vi "MasterAquisitionFile_2P.vi"() -> ()   [LabVIEW 2017]
uses:
  <vilib>/userdefined/High Color/IMAQdx.ctl
  <vilib>/vision/driver/IMAQdx.llb/IMAQdx Camera Control Mode.ctl
  <vilib>/vision/driver/IMAQdx.llb/IMAQdx Acquisition Mode.ctl
  <vilib>/vision/driver/IMAQdx.llb/IMAQdx Buffer Number Mode.ctl
  <vilib>/DAQmx/miscellaneous.llb/DAQmx Fill In Error Info.vi
  <vilib>/DAQmx/read.llb/DAQmx Read (Digital 1D Bool 1Chan 1Samp).vi
  <vilib>/DAQmx/create/channels.llb/DAQmx Create Channel (DI-Digital Input).vi
  <vilib>/DAQmx/create/channels.llb/DAQmx Create Channel (DO-Digital Output).vi
  <vilib>/DAQmx/read.llb/DAQmx Read (Analog 1D Wfm NChan NSamp).vi
  <vilib>/DAQmx/configure/trigger.llb/DAQmx Start Trigger (Digital Edge).vi
  <vilib>/DAQmx/configure/timing.llb/DAQmx Timing (Sample Clock).vi
  <vilib>/DAQmx/create/channels.llb/DAQmx Create Channel (AI-Voltage-Basic).vi
  <vilib>/DAQmx/configure/timing.llb/DAQmx Timing (Implicit).vi
  <vilib>/DAQmx/create/channels.llb/DAQmx Create Channel (CO-Pulse Generation-Frequency).vi
  <vilib>/DAQmx/write.llb/DAQmx Write (Digital 1D Bool NChan 1Samp 1Line).vi
  <vilib>/vision/driver/NI_Vision_Acquisition_Software.lvlib
  <resource>/objmgr/imaqdx.rc
panel:
  in  "stop":bool
  in  "Offset (s)":dbl=15.0
  in  "Duration (s)":dbl=0.1 step=0.1
  in  "Interval (s)":dbl=30.0
  out "Solenoids":bool[](array[boolean])
  in  "Left Pad Solenoid":tag="Dev1/port0/line5"
  in  "Right Pad Solenoid":tag="Dev1/port0/line6"
  in  "Auditory Solenoid":tag="Dev1/port0/line7"
  in  "RPad":dbl=1.0
  in  "LPad":dbl=1.0
  in  "Aud":dbl=1.0
  out "?":T1(plugin-control)
  out "Web Cam Fs":dbl(knob) scale=0.0..200.0
  out "Web Cam":bool
  in  "WebCam ID":T2="cam2"
  out "Complete":bool
  out "Whisk Cam":bool
  out "Analog":bool
  out "MScan Trig":bool
  in  "MScan Trigger":tag="Dev1/port0/line3"
  out "?":bool[](array[boolean])
  out "Hexadecimal Data":u32 format="%x"
  out "Time Elapsed (Min)":cluster{dbl, dbl}(slide)={16.0, 0.0} scale=0.0..16.0 scale format="%#_2g"
  out "Whisker Camera":bool=TRUE
  out "Analog Data":bool
  out "Analog Samples":i32
  in  "Analog Channel Labels":string[](array[string])=["Force_Sensor", "Force_Sensor", "Solenoid_LeftPad", "Solenoid_RightPad", "Solenoid_Auditory", "Respiration", "EMG", "Neural_RH"]
  in  "Analog Input Channels":tag="Dev1/ai2"
  in  "Whisker Cam ID":T2="cam1"
  in  "?":cluster{"Analog Fs":u16}={"Analog Fs"=20000} {"Analog Fs" format="%0.0f"}
  in  "?":cluster{"WhiskerCam Fs":u16}={"WhiskerCam Fs"=150}
  out "Notes Size":i32=7
  out "Notes Reversed":string[](array[string])=["Experimenter", "Animal ID", "Isoflurane time", "Amplifier Gain", "Session ID", "Hemisphere", "Solenoid PSI"]
  out "Notes Array":string[](array[string])=["Solenoid PSI", "Hemisphere", "Session ID", "Amplifier Gain", "Isoflurane time", "Animal ID", "Experimenter"]
  in  "Notes:":T3={"Experimenter"="0\n", "Animal ID"="", "Isoflurane time"="", "Amplifier Gain"="", "Session ID"="", "Hemisphere"="", "Solenoid PSI"=""}
  in  "Whisk Cam Trigger":tag="Dev1/ctr0"
  in  "Target Path":path=path "C:/Users/klt8/Documents" caption="Final Saved File Location"
  out "Dropped":u32(slide) caption="Whisk Cam" scale=0.0..50.0
  out "Current File Name":string="190410_10_32_56"
  in  "Time (min)":dbl(knob)=16.0 min=0.5 max=20.0 step=0.5 scale=0.0..20.0 scale format="%#_3g"
  in  "Temp Path":path=path "C:/LabVIEW Temp Files" caption="Temporary File Path"
  out "Last Whisk Buffer":u32=45000
  out "Whisk Cam Fs":dbl(knob) scale=0.0..200.0 scale format="%#1_6g"
  # "LPad Sol"
  # "RPad Sol"
  # "Aud Sol"
  # "Web Cam ID"
  # "Whisk Cam ID"
  # "AnalogFs"
  # "WhiskFs"
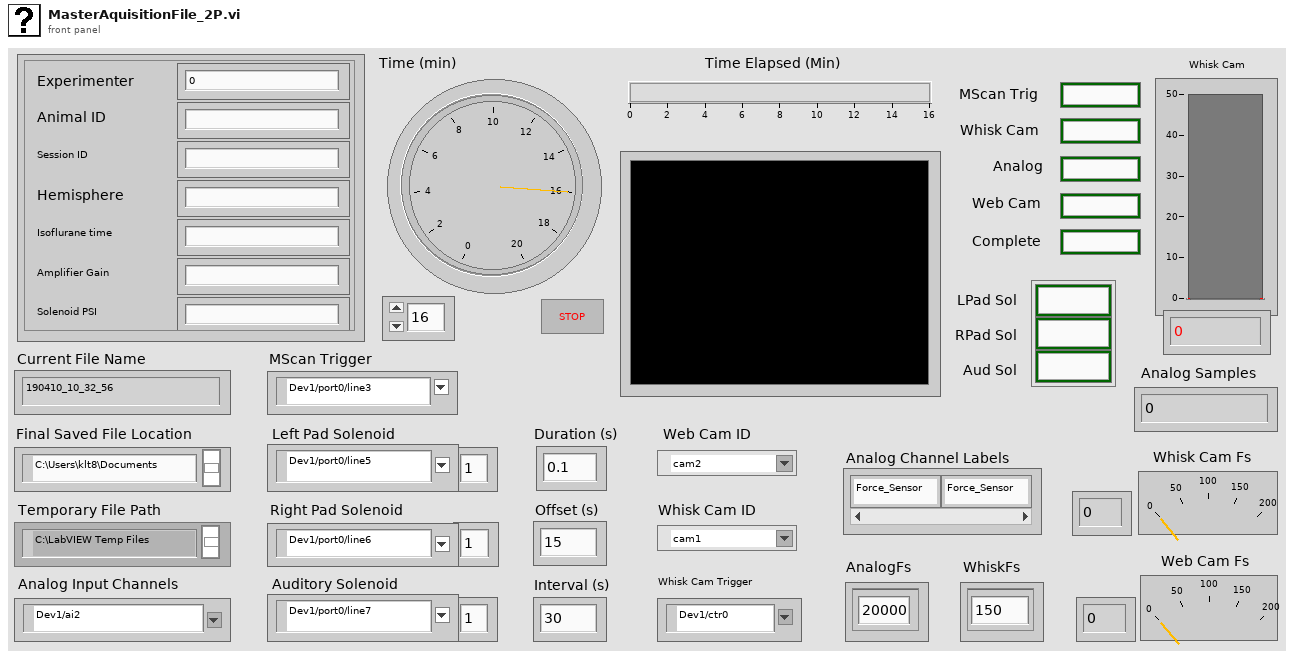
[diagram p1: front panel]
types:
  T1 = typedef "IMAQ Image.ctl" = refnum<image>
  T2 = typedef "IMAQdx.ctl" = refnum<k21>
  T3 = cluster{"Experimenter":string, "Animal ID":string, "Isoflurane time":string, "Amplifier Gain":string, "Session ID":string, "Hemisphere":string, "Solenoid PSI":string}
  T4 = enum16{"open", "open or create", "create or replace", "create", "open (read-only)"}
  T5 = typedef "NI_Vision_Acquisition_Software.lvlib/IMAQdx Camera Control Mode.ctl" = enum32{"Controller", "Listener"}
  T6 = enum16{"open", "replace", "create", "open or create", "replace or create", "replace or create with confirmation"}
  T7 = typedef "NI_Vision_Acquisition_Software.lvlib/IMAQdx Acquisition Mode.ctl" = enum32{"One Shot", "Continuous"}
  T8 = enum16{"big-endian, network order", "native, host order", "little-endian"}
  T9 = typedef "NI_Vision_Acquisition_Software.lvlib/IMAQdx Buffer Number Mode.ctl" = enum32{"Next", "Last", "Buffer Number", "Every", "Last New"}
  T10 = typedef "Image Type" = u32
  T11 = typedef "IMAQ AVI2 Refnum.ctl" = refnum<k20>
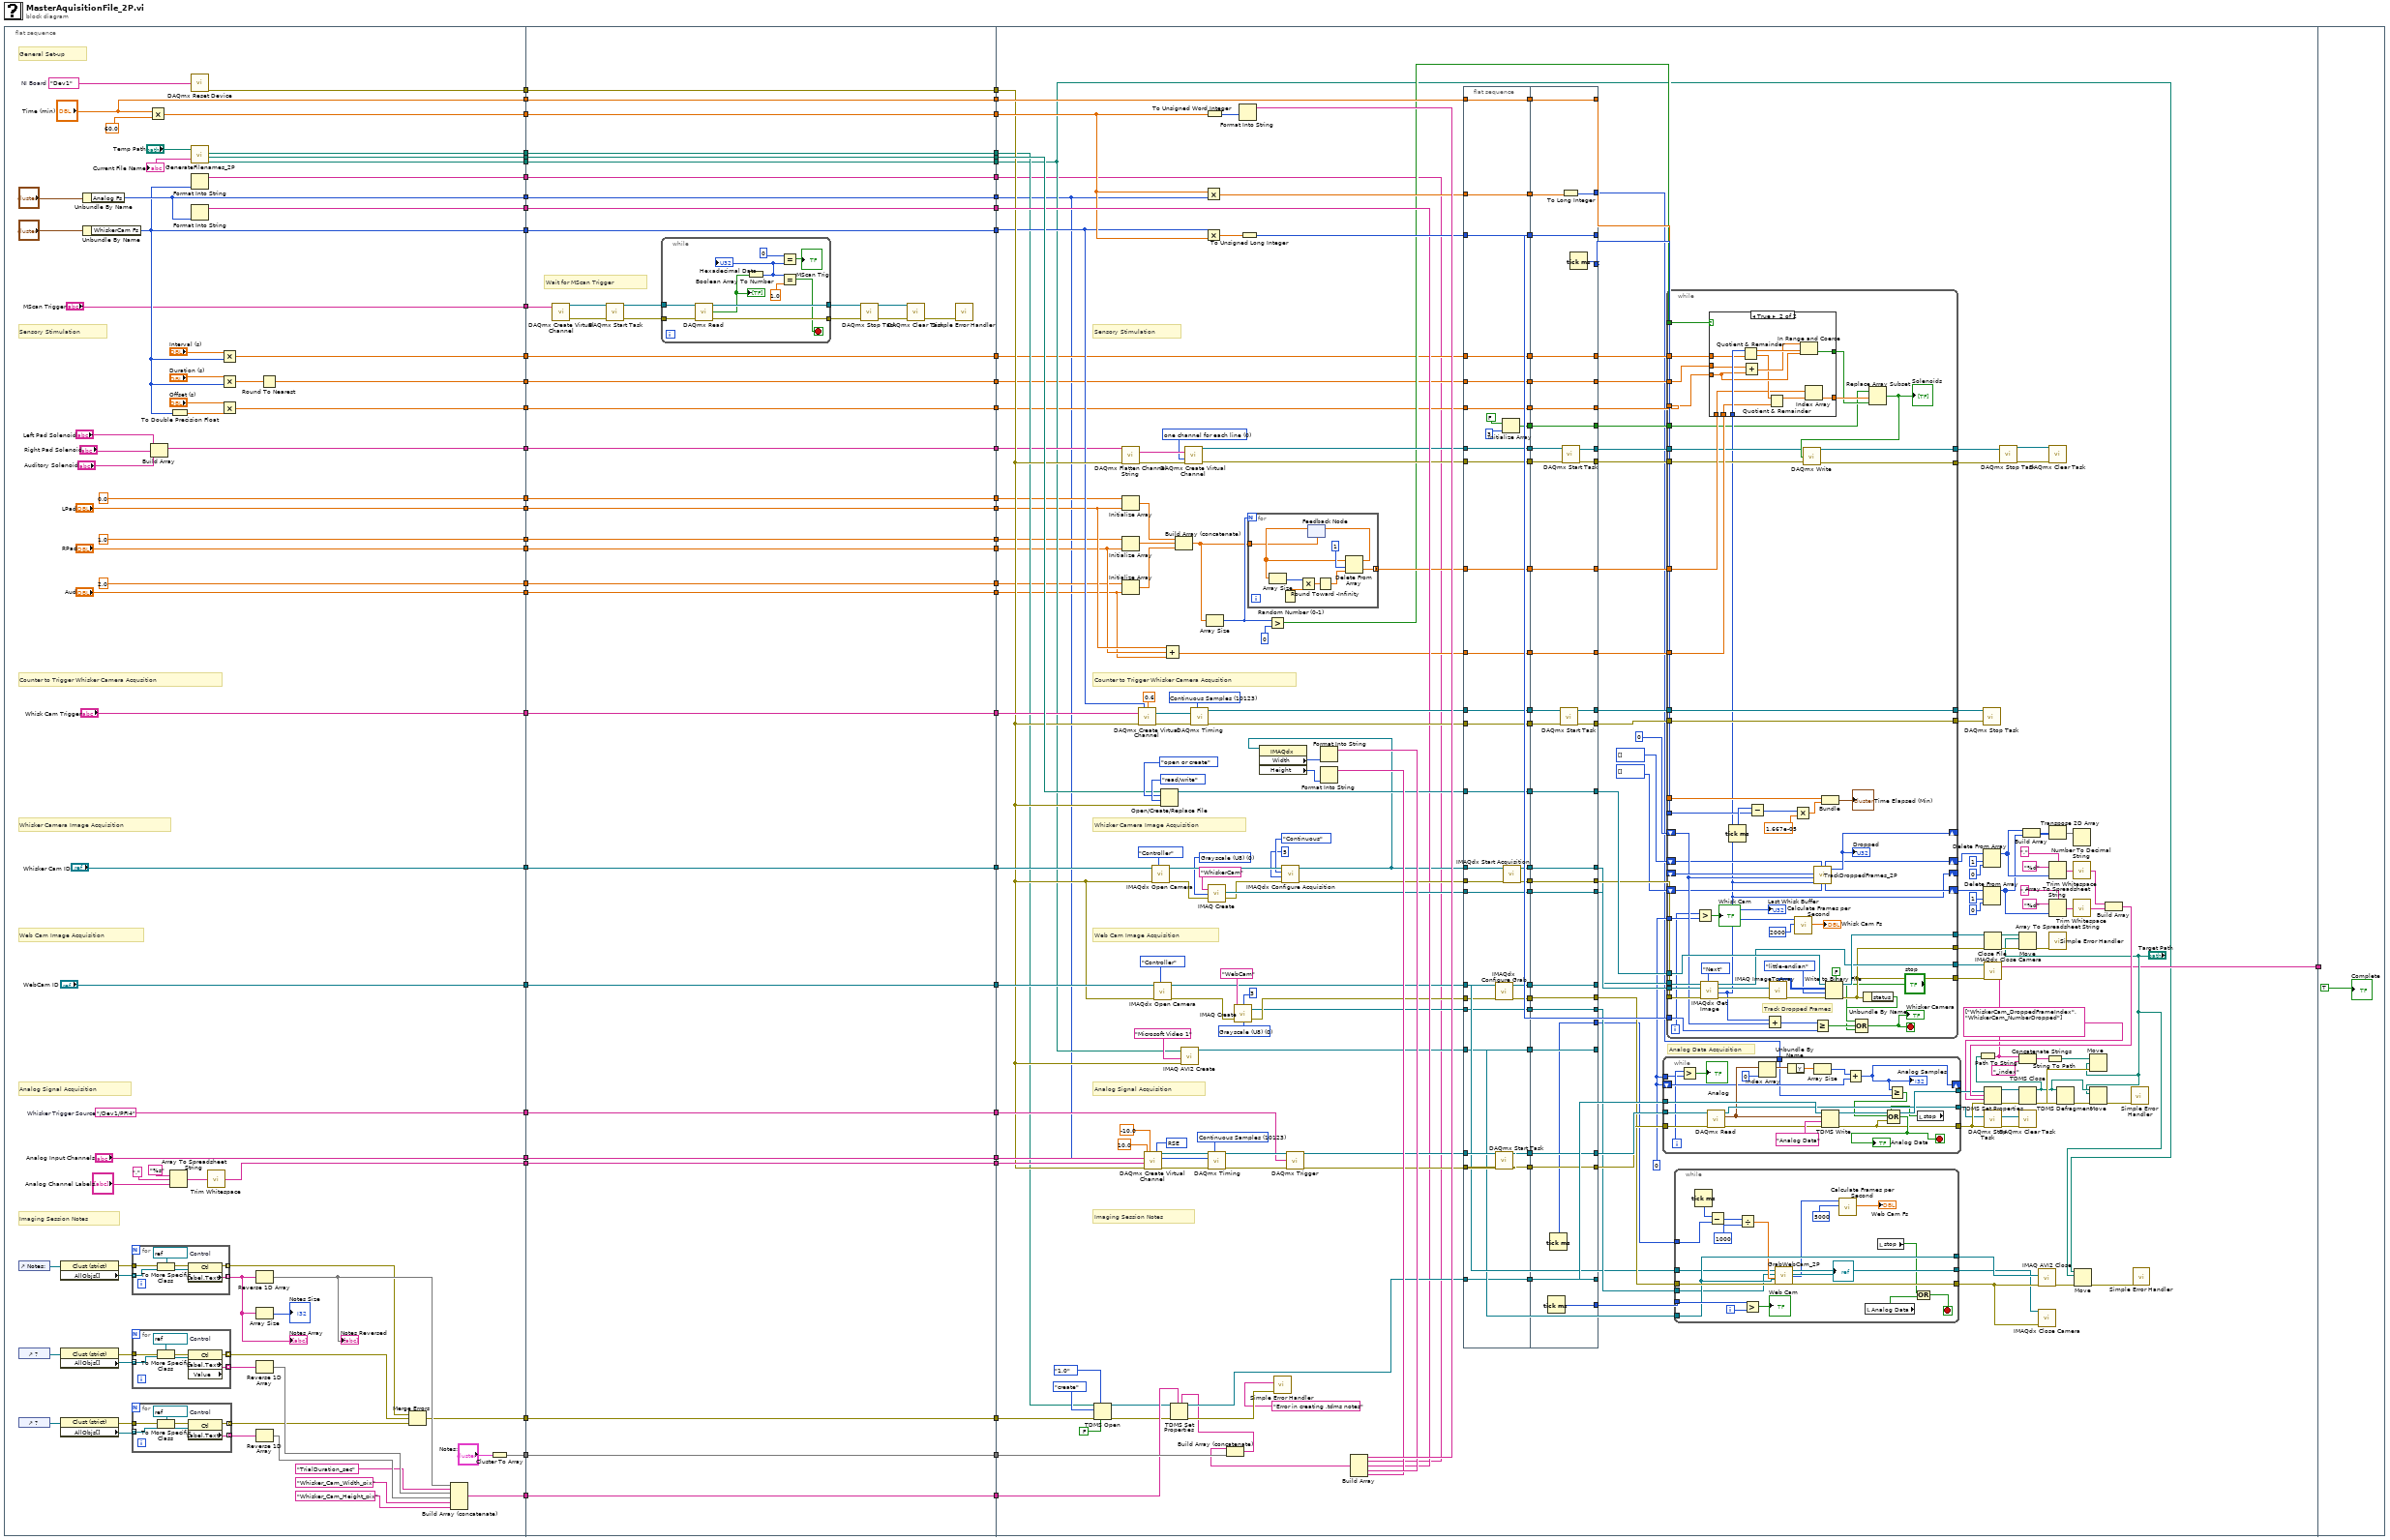
[diagram p0: block diagram]
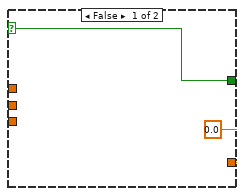
[diagram p2: hidden frame]
diagram:
  n1 = flat-sequence {
    tunnel: [w100] -> w45
    tunnel: [w99] -> w44
    tunnel: ["Time (min)"] -> w43
    tunnel: [w97] -> w42
    tunnel: [w96] -> w41
    tunnel: [w95] -> w40
    tunnel: [w94] -> w39
    tunnel: [w93] -> w38
    tunnel: ["Whisk Cam Trigger"] -> w37
    tunnel: [w91] -> w36
    tunnel: ["Analog Input Channels"] -> w35
    tunnel: ["Whisker Cam ID"] -> w34
    tunnel: [w88] -> w33
    tunnel: [w84] -> w32
    tunnel: [w87] -> w31
    tunnel: ["WebCam ID"] -> w29
    tunnel: ["MScan Trigger"] -> w28
    tunnel: [w81] -> w27
    tunnel: [w80] -> w24
    tunnel: [w79] -> w23
    tunnel: [w75] -> w19
    tunnel: [w70] -> w15
    tunnel: [w69] -> w14
    tunnel: [w68] -> w13
    tunnel: [1.0 ("element")] -> w6
    tunnel: [0.0 ("element")] -> w5
    tunnel: [2.0 ("element")] -> w4
    tunnel: ["Aud"] -> w3
    tunnel: ["RPad"] -> w2
    tunnel: ["LPad"] -> w1
    tunnel: [w168] -> w60
    tunnel: [w180] -> w59
    tunnel: [w181] -> w58
    tunnel: [w182] -> w57
    tunnel: [w183] -> w56
    tunnel: [w170] -> w55
    tunnel: [w184] -> w54
    tunnel: [w169] -> w53
    tunnel: [w185] -> w52
    tunnel: [w186] -> w51
    tunnel: [w187] -> w50
    tunnel: [w188] -> w49
    tunnel: [w189] -> w48
    tunnel: [w190] -> w47
    tunnel: [w191] -> w46
    tunnel: w45 -> [w191]
    tunnel: w44 -> [w190]
    tunnel: w43 -> [w189]
    tunnel: w42 -> [w188]
    tunnel: w41 -> [w187]
    tunnel: w40 -> [w186]
    tunnel: w39 -> [w185]
    tunnel: w38 -> [w169]
    tunnel: w37 -> [w184]
    tunnel: w36 -> [w170]
    tunnel: w35 -> [w183]
    tunnel: w34 -> [w182]
    tunnel: w33 -> [w181]
    tunnel: w32 -> [w180]
    tunnel: w31 -> [w168]
    tunnel: [w166] -> w30
    tunnel: w29 -> [w166]
    tunnel: w28 -> [w167]
    tunnel: w27 -> [w165]
    tunnel: [w165] -> w26
    tunnel: w24 -> [w164]
    tunnel: w23 -> [w163]
    tunnel: [w164] -> w22
    tunnel: [w163] -> w21
    tunnel: [w162] -> w20
    tunnel: w19 -> [w162]
    tunnel: [w161] -> w18
    tunnel: [w159] -> w17
    tunnel: [w160] -> w16
    tunnel: w15 -> [w161]
    tunnel: w14 -> [w160]
    tunnel: w13 -> [w159]
    tunnel: [w153] -> w12
    tunnel: [w154] -> w11
    tunnel: [w155] -> w10
    tunnel: [w158] -> w9
    tunnel: [w157] -> w8
    tunnel: [w156] -> w7
    tunnel: w6 -> [w158]
    tunnel: w5 -> [w157]
    tunnel: w4 -> [w156]
    tunnel: w3 -> [w155]
    tunnel: w2 -> [w154]
    tunnel: w1 -> [w153]
    tunnel: w60 -> [w297]
    tunnel: w59 -> [w307]
    tunnel: w58 -> [w256]
    tunnel: w57 -> [w306]
    tunnel: w56 -> [w305]
    tunnel: w55 -> [w304]
    tunnel: w54 -> [w303]
    tunnel: w53 -> [w302]
    tunnel: w52 -> [w240]
    tunnel: w51 -> [w206]
    tunnel: w50 -> [w301]
    tunnel: w49 -> [w205]
    tunnel: w48 -> [w292]
    tunnel: w47 -> [w300]
    tunnel: w46 -> [w299]
    tunnel: w30 -> [w283]
    tunnel: w26 -> [w218]
    tunnel: [w229] -> w25
    tunnel: w22 -> [w224]
    tunnel: w21 -> [w222]
    tunnel: w20 -> [w219]
    tunnel: w18 -> [w217]
    tunnel: w17 -> [w208]
    tunnel: w16 -> [w216]
    tunnel: w12 -> [w215]
    tunnel: w11 -> [w214]
    tunnel: w10 -> [w213]
    tunnel: w9 -> [w212]
    tunnel: w8 -> [w211]
    tunnel: w7 -> [w210]
    tunnel: w25 -> [_]
    frame #0 {
      w100 = tag "/Dev1/PFI4"  # Whisker Trigger Source
      w104 = tag "Dev1"  # NI Board
      # "Sensory Stimulation"
      # "General Set-up"
      # "Whisker Camera Image Acquisition"
      # "Imaging Session Notes"
      # "Counter to Trigger Whisker Camera Acqusition"
      # "Web Cam Image Acquisition"
      # "Analog Signal Acquisition"
      n2 = control-ref of="Notes:"() -> (w117:refnum<vi>)
      n3 = control-ref of="?"() -> (w115:refnum<vi>)
      n4 = control-ref of="?"() -> (w108:refnum<vi>)
      n5 = property class="Clust (strict)"(reference=w117) -> (error out=w116:errorcluster, "AllObjs[]"=w118:refnum<vi>[])  [unwired: 1 in, 1 out]
      n6 = property class="Clust (strict)"(reference=w115) -> (error out=w113:errorcluster, "AllObjs[]"=w114:refnum<vi>[])  [unwired: 1 in, 1 out]
      n7 = property class="Clust (strict)"(reference=w108) -> (error out=w109:errorcluster, "AllObjs[]"=w111:refnum<vi>[])  [unwired: 1 in, 1 out]
      n8 = Unbundle By Name("?") -> ("Analog Fs"=w95:u16)
      n9 = Unbundle By Name("?") -> ("WhiskerCam Fs"=w94:u16)
      n10 = for {
        tunnel: [w136] -> w123 mode=indexing
        tunnel: w118 -> [w135] mode=indexing
        tunnel: w116 -> [w134]
        tunnel: [w132] -> w122 mode=indexing
        w137 = refnum<vi> refnum  # Control
        n11 = To More Specific Class(target class=w137, reference=w135, error in=w134) -> (specific class reference=w138:refnum<vi>, error out=w133:errorcluster)
        n12 = property class="Ctl"(reference=w138, error in=w133) -> (error out=w132:errorcluster, "Label.Text"=w136:string)  [unwired: 1 out]
      }
      "Notes Array" <- w123
      n13 = for {
        tunnel: [w143] -> w112 mode=indexing
        tunnel: w114 -> [w142] mode=indexing
        tunnel: w113 -> [w141]
        tunnel: [w139] -> w121 mode=indexing
        w144 = refnum<vi> refnum  # Control
        n14 = To More Specific Class(target class=w144, reference=w142, error in=w141) -> (specific class reference=w145:refnum<vi>, error out=w140:errorcluster)
        n15 = property class="Ctl" props=["Label", "Text", "Value"](reference=w145, error in=w140) -> (error out=w139:errorcluster, "Label.Text"=w143:string)  [unwired: 2 out]
      }
      n16 = for {
        tunnel: [w150] -> w110 mode=indexing
        tunnel: w111 -> [w149] mode=indexing
        tunnel: w109 -> [w148]
        tunnel: [w146] -> w120 mode=indexing
        w151 = refnum<vi> refnum  # Control
        n17 = To More Specific Class(target class=w151, reference=w149, error in=w148) -> (specific class reference=w152:refnum<vi>, error out=w147:errorcluster)
        n18 = property class="Ctl"(reference=w152, error in=w147) -> (error out=w146:errorcluster, "Label.Text"=w150:string)  [unwired: 1 out]
      }
      n19 = Multiply(x="Time (min)", y=60.0) -> (x*y=w99:dbl)
      n20 = Build Array("Left Pad Solenoid", "Right Pad Solenoid", "Auditory Solenoid") -> (w75:tag[])
      n21 = Array To Spreadsheet String(delimiter (Tab)=",", array="Analog Channel Labels", 3:"%s" ("format string")) -> (spreadsheet string=w125:string)
      n22 = To Double Precision Float(number=w94) -> (double precision float=w74:dbl)
      n23 = call <vilib>:"DAQmx Reset Device.vi"("device in"=w104) -> ("error out"=w88:errorcluster)  [unwired: 14 in]
      n24 = call "GenerateFilenames_2P.vi"("path"="Temp Path") -> ("Analog file name"=→"Current File Name":string, "TDMS Path"=w79:path, "Basler Path"=w84:path, "WebCam Path"=w81:path)  [unwired: 6 in]
      n25 = Format Into String(w94) -> (resulting string=w97:string)  [unwired: 3 in, 1 out]
      n26 = Format Into String(w95) -> (resulting string=w96:string)  [unwired: 3 in, 1 out]
      n27 = call <vilib>:"Trim Whitespace.vi"("string"=w125) -> ("trimmed string"=w91:string)  [unwired: 1 in]
      n28 = Multiply(x="Interval (s)", y=w94) -> (x*y=w68:dbl)
      n29 = Multiply(x="Duration (s)", y=w94) -> (x*y=w67:dbl)
      n30 = Multiply(x="Offset (s)", y=w74) -> (x*y=w70:dbl)
      n31 = Reverse 1D Array(array=w123) -> (reversed array=w124:string[])
      "Notes Reversed" <- w124
      n32 = Array Size(array=w123) -> (size(s)=→"Notes Size":i32)
      n33 = Reverse 1D Array(array=w112) -> (reversed array=w130:string[])
      n34 = Reverse 1D Array(array=w110) -> (reversed array=w131:string[])
      n35 = Round To Nearest(number=w67) -> (nearest integer value=w69:dbl)
      n36 = Merge Errors(w122, w121, w120) -> (w80:errorcluster)
      n37 = Build Array (concatenate)(w124, "TrialDuration_sec", w130, w131, "Whisker_Cam_Width_pix", "Whisker_Cam_Height_pix") -> (w87:string[])
      n38 = Cluster To Array(cluster="Notes:") -> (array=w93:string[])
    }
    frame #1 {
      # "Wait for MScan Trigger"
      n39 = call-poly <vilib>:"DAQmx Create Virtual Channel.vi"("lines"=w167) -> ("task out"=w175:refnum<k21>, "error out"=w176:errorcluster)  [unwired: 13 in]
      n40 = call <vilib>:"DAQmx Start Task.vi"("task/channels in"=w175, "error in"=w176) -> ("task out"=w179:refnum<k21>, "error out"=w178:errorcluster)  [unwired: 12 in]
      n41 = while {
        tunnel: w179 -> [w201]
        tunnel: w178 -> [w200]
        tunnel: [w198] -> w173
        tunnel: [w199] -> w174
        stop <- w193 stop-if-true
        n42 = call-poly <vilib>:"DAQmx Read.vi"("task/channels in"=w201, "error in"=w200) -> ("task out"=w199:refnum<k21>, "data"=w197:bool[], "error out"=w198:errorcluster)  [unwired: 11 in]
        "?" <- w197
        n43 = Boolean Array To Number(Boolean array=w197) -> (number=w192:u32)
        "Hexadecimal Data" <- w192
        n44 = Equal?(x=w192, y=u32 0) -> (x = y?=→"MScan Trig":bool)
        n45 = Equal?(x=w192, y=1.0) -> (x = y?=w193:bool)
      }
      n46 = call <vilib>:"DAQmx Stop Task.vi"("task/channels in"=w174, "error in"=w173) -> ("task out"=w172:refnum<k21>, "error out"=w171:errorcluster)  [unwired: 12 in]
      n47 = call <vilib>:"DAQmx Clear Task.vi"("task in"=w172, "error in"=w171) -> ("error out"=w177:errorcluster)  [unwired: 13 in]
      n48 = call <vilib>:"Simple Error Handler.vi"("error in (no error)"=w177) -> ()  [unwired: 4 in, 5 out]
    }
    frame #2 {
      w209 = 0 items=["one channel for each line", "one channel for all lines"] ("line grouping")
      w287 = T10 0 items=["Grayscale (U8)", "Grayscale (I16)", "Grayscale (SGL)", "Complex (CSG)", "RGB (U32)", "HSL (U32)", "RGB (U64)", "Grayscale (U16)"] ("Image Type")
      w271 = u32 0 ("y")
      w316 = 10123 items=["Finite Samples"=10178, "Continuous Samples"=10123, "Hardware Timed Single Point"=12522] ("sample mode")
      w315 = 10083 items=["default"=-1, "RSE"=10083, "NRSE"=10078, "Differential"=10106, "Pseudodifferential"=12529] ("input terminal configuration")
      w317 = 10123 items=["Finite Samples"=10178, "Continuous Samples"=10123, "Hardware Timed Single Point"=12522] ("sample mode")
      w313 = T10 0 items=["Grayscale (U8)", "Grayscale (I16)", "Grayscale (SGL)", "Complex (CSG)", "RGB (U32)", "HSL (U32)", "RGB (U64)", "Grayscale (U16)"] ("Image Type")
      # "Sensory Stimulation"
      # "Whisker Camera Image Acquisition"
      # "Imaging Session Notes"
      # "Counter to Trigger Whisker Camera Acqusition"
      # "Web Cam Image Acquisition"
      # "Analog Signal Acquisition"
      # "Analog Data Acquisition"
      n49 = TDMS Open(6:FALSE ("disable buffering? (T)"), 7:enum16{"1.0", "2.0"}."1.0" ("file format version (2.0)"), 8:w224, 10:T4."create" ("operation (0:open)"), 11:w222) -> (0:w221:errorcluster, 3:w220:refnum<k34>)  [unwired: 2 in]
      n50 = call <vilib>:"DAQmx Flatten Channel String.vi"("names in"=w219, "error in"=w256) -> ("names out"=w261:string, "error out"=w262:errorcluster)  [unwired: 12 in]
      n51 = Initialize Array(w211, w215) -> (w258:dbl[])
      n52 = Initialize Array(w212, w214) -> (w259:dbl[])
      n53 = Initialize Array(w210, w213) -> (w228:dbl[])
      n54 = call-poly <vilib>:"DAQmx Create Virtual Channel.vi"("frequency"=w240, "duty cycle"=0.6, "counter"=w303, "error in"=w256) -> ("task out"=w340:refnum<k21>, "error out"=w341:errorcluster)  [unwired: 10 in]
      n55 = call-poly <vilib>:"DAQmx Create Virtual Channel.vi"("maximum value"=10.0, "minimum value"=-10.0, "input terminal configuration"=w315, "physical channels"=w305, "name to assign"=w304, "error in"=w256) -> ("task out"=w349:refnum<k21>, "error out"=w350:errorcluster)  [unwired: 8 in]
      n56 = call <vilib>:"IMAQdx Open Camera.vi"("Camera Control Mode"=IMAQdx_Camera_Control_Mode."Controller", "error in"=w256, "Session In"=w306) -> ("error out"=w338:errorcluster, "Session Out"=w337:T2)  [unwired: 7 in]
      n57 = call <vilib>:"IMAQdx Open Camera.vi"("Camera Control Mode"=IMAQdx_Camera_Control_Mode."Controller", "error in"=w256, "Session In"=w283) -> ("error out"=w284:errorcluster, "Session Out"=w282:T2)  [unwired: 7 in]
      n58 = Open/Create/Replace File(file path (use dialog)=w307, error in=w256, operation (0:open)=T6."open or create", access (0:read/write)=enum16{"read/write", "read-only", "write-only"}."read/write") -> (refnum out=w348:refnum<file>)  [unwired: 2 in, 2 out]
      n59 = Compound Arithmetic op=ADD(w215, w214, w213) -> (w248:dbl)
      n60 = Build Array (concatenate)(w258, w259, w228) -> (w260:dbl[])
      n61 = call "IMAQ AVI2 Create"("error in (no error)"=w256, "Codec"="Microsoft Video 1", "AVI Path"=w218) -> ("AVI Refnum"=w266:T11)  [unwired: 7 in, 1 out]
      n62 = call-poly <vilib>:"DAQmx Create Virtual Channel.vi"("lines"=w261, "line grouping"=w209, "error in"=w262) -> ("task out"=w255:refnum<k21>, "error out"=w252:errorcluster)  [unwired: 11 in]
      n63 = call-poly <vilib>:"DAQmx Timing.vi"("task/channels in"=w340, "sample mode"=w317, "error in"=w341) -> ("task out"=w359:refnum<k21>, "error out"=w360:errorcluster)  [unwired: 11 in]
      n64 = Multiply(x=w300, y=w206) -> (x*y=w391:dbl)
      n65 = Multiply(x=w240, y=w300) -> (x*y=w392:dbl)
      n66 = To Unsigned Word Integer(number=w300) -> (unsigned 16bit integer=w376:u16)
      n67 = Array Size(array=w260) -> (size(s)=w263:i32)
      n68 = call "IMAQ Create"("Image Name"="WhiskerCam", "Image Type"=w313, "error in (no error)"=w338) -> ("New Image"=w379:T1, "error out"=w339:errorcluster)  [unwired: 2 in]
      n69 = call-poly <vilib>:"DAQmx Timing.vi"("task/channels in"=w349, "sample mode"=w316, "rate"=w206, "error in"=w350) -> ("task out"=w351:refnum<k21>, "error out"=w352:errorcluster)  [unwired: 10 in]
      n70 = call "IMAQ Create"("Border Size"=3, "Image Name"="WebCam", "Image Type"=w287, "error in (no error)"=w284) -> ("New Image"=w280:T1, "error out"=w281:errorcluster)  [unwired: 1 in]
      n71 = Format Into String(w376) -> (resulting string=w401:string)  [unwired: 3 in, 1 out]
      n72 = To Unsigned Long Integer(number=w392) -> (unsigned 32bit integer=w393:u32)
      n73 = for {
        N: w263 -> [_]
        tunnel: w260 -> [w413]
        tunnel: [w414] -> w250 mode=concatenating
        n74 = Random Number (0-1)() -> (number: 0 to 1=w420:dbl)
        n75 = feedback #1(w413) -> (w416:dbl[])
        n76 = Array Size(array=w416) -> (size(s)=w421:i32)
        n77 = Multiply(x=w421, y=w420) -> (x*y=w419:dbl)
        n78 = Round Toward -Infinity(1:w419) -> (0:w418:dbl)
        n79 = Delete From Array(array=w416, length=1, index=w418) -> (deleted portion=w414:dbl[], array with subset deleted=w415:dbl[])
        n80 = feedback-in #1(w415) -> ()
      }
      n81 = Greater?(x=w263, y=0) -> (0:w247:bool)
      n82 = call <vilib>:"IMAQdx Configure Acquisition.vi"("error in"=w339, "Number of Buffers"=u32 5, "Continuous?"=IMAQdx_Acquisition_Mode."Continuous", "Session In"=w337) -> ("error out"=w343:errorcluster, "Session Out"=w207:T2)  [unwired: 6 in]
      n83 = property class="IMAQdx"(reference=w207) -> ("Width"=w377:u32, "Height"=w378:u32)  [unwired: 1 in, 2 out]
      n84 = call-poly <vilib>:"DAQmx Trigger.vi"("task/channels in"=w351, "source"=w299, "error in"=w352) -> ("task out"=w353:refnum<k21>, "error out"=w354:errorcluster)  [unwired: 11 in]
      n85 = Format Into String(w377) -> (resulting string=w400:string)  [unwired: 3 in, 1 out]
      n86 = Format Into String(w378) -> (resulting string=w399:string)  [unwired: 3 in, 1 out]
      n87 = Build Array(w401, w205, w301, w400, w399) -> (w202:string[])
      n88 = Build Array (concatenate)(w302, w202) -> (w308:string[])
      n89 = TDMS Set Properties(5:w308, 7:w297, 8:w221, 11:w220) -> (0:w375:errorcluster, 3:w374:refnum<k34>)  [unwired: 2 in, 2 out]
      n90 = call <vilib>:"Simple Error Handler.vi"("error source (\" \")"="Error in creating .tdms notes" ("error source (\" \")"), "error in (no error)"=w375) -> ()  [unwired: 3 in, 5 out]
      n91 = flat-sequence {
        tunnel: w207 -> [w496]
        tunnel: w343 -> [w495]
        tunnel: [w494] -> w412
        tunnel: [w493] -> w411
        tunnel: [w492] -> w410
        tunnel: w379 -> [w492]
        tunnel: [w491] -> w409
        tunnel: w348 -> [w491]
        tunnel: w353 -> [w490]
        tunnel: w354 -> [w489]
        tunnel: [w488] -> w408
        tunnel: [w487] -> w407
        tunnel: [w486] -> w406
        tunnel: w374 -> [w486]
        tunnel: w359 -> [w485]
        tunnel: [w485] -> w405
        tunnel: w360 -> [w484]
        tunnel: [w484] -> w404
        tunnel: w391 -> [w483]
        tunnel: [w483] -> w403
        tunnel: w393 -> [w482]
        tunnel: [w482] -> w402
        tunnel: w292 -> [w481]
        tunnel: [w481] -> w291
        tunnel: w282 -> [w480]
        tunnel: w281 -> [w479]
        tunnel: w280 -> [w478]
        tunnel: [w478] -> w279
        tunnel: [w477] -> w278
        tunnel: [w476] -> w277
        tunnel: [w475] -> w267
        tunnel: w266 -> [w475]
        tunnel: w255 -> [w474]
        tunnel: [w474] -> w254
        tunnel: w252 -> [w473]
        tunnel: [w473] -> w253
        tunnel: [w472] -> w251
        tunnel: w250 -> [w472]
        tunnel: [w471] -> w249
        tunnel: w248 -> [w471]
        tunnel: [w466] -> w244
        tunnel: [w465] -> w242
        tunnel: [w467] -> w239
        tunnel: [w468] -> w231
        tunnel: w217 -> [w467]
        tunnel: w208 -> [w466]
        tunnel: w216 -> [w465]
        tunnel: [w521] -> w295
        tunnel: [w520] -> w296
        tunnel: [w528] -> w344
        tunnel: w412 -> [w528]
        tunnel: [w527] -> w345
        tunnel: w411 -> [w527]
        tunnel: [w526] -> w346
        tunnel: w410 -> [w526]
        tunnel: [w525] -> w347
        tunnel: w409 -> [w525]
        tunnel: [w524] -> w356
        tunnel: w408 -> [w524]
        tunnel: [w523] -> w355
        tunnel: w407 -> [w523]
        tunnel: [w522] -> w357
        tunnel: w406 -> [w522]
        tunnel: w405 -> [w517]
        tunnel: w404 -> [w519]
        tunnel: w403 -> [w498]
        tunnel: w402 -> [w518]
        tunnel: [w518] -> w398
        tunnel: [w516] -> w336
        tunnel: w291 -> [w515]
        tunnel: [w515] -> w290
        tunnel: [w514] -> w270
        tunnel: w279 -> [w514]
        tunnel: [w513] -> w268
        tunnel: w278 -> [w513]
        tunnel: [w512] -> w269
        tunnel: w277 -> [w512]
        tunnel: [w511] -> w227
        tunnel: w267 -> [w510]
        tunnel: [w510] -> w265
        tunnel: w254 -> [w509]
        tunnel: w253 -> [w508]
        tunnel: w251 -> [w507]
        tunnel: [w507] -> w246
        tunnel: w249 -> [w506]
        tunnel: [w506] -> w245
        tunnel: w244 -> [w505]
        tunnel: [w505] -> w243
        tunnel: [w504] -> w241
        tunnel: w242 -> [w504]
        tunnel: [w503] -> w238
        tunnel: w239 -> [w503]
        tunnel: [w502] -> w237
        tunnel: [w501] -> w236
        tunnel: [w500] -> w230
        tunnel: w231 -> [w500]
        tunnel: [w499] -> w226
        tunnel: [w497] -> w204
        frame #0 {
          n92 = call <vilib>:"IMAQdx Configure Grab.vi"("error in"=w479, "Session In"=w480) -> ("error out"=w476:errorcluster, "Session Out"=w477:T2)  [unwired: 8 in]
          n93 = call <vilib>:"DAQmx Start Task.vi"("task/channels in"=w490, "error in"=w489) -> ("task out"=w488:refnum<k21>, "error out"=w487:errorcluster)  [unwired: 12 in]
          n94 = Initialize Array(FALSE, 3 ("dimension size")) -> (w468:bool[])
          n95 = call <vilib>:"IMAQdx Start Acquisition.vi"("error in"=w495, "Session In"=w496) -> ("error out"=w493:errorcluster, "Session Out"=w494:T2)  [unwired: 8 in]
        }
        frame #1 {
          n96 = Tick Count (ms)() -> (millisecond timer value=w511:u32)
          n97 = Tick Count (ms)() -> (millisecond timer value=w499:u32)
          n98 = call <vilib>:"DAQmx Start Task.vi"("task/channels in"=w517, "error in"=w519) -> ("task out"=w521:refnum<k21>, "error out"=w520:errorcluster)  [unwired: 12 in]
          n99 = To Long Integer(number=w498) -> (32bit integer=w497:i32)
          n100 = call <vilib>:"DAQmx Start Task.vi"("task/channels in"=w509, "error in"=w508) -> ("task out"=w502:refnum<k21>, "error out"=w501:errorcluster)  [unwired: 12 in]
          n101 = Tick Count (ms)() -> (millisecond timer value=w516:u32)
        }
      }
      n102 = while {
        tunnel: w355 -> [w464]
        tunnel: w356 -> [w463]
        tunnel: w357 -> [w462]
        tunnel: [w461] -> w380
        tunnel: [w449] -> w381
        tunnel: [w460] -> w358
        shift-right: [w453] -> _
        shift-left: w271 -> [w454]
        tunnel: w271 -> [w445]
        tunnel: w204 -> [w443]
        i -> [w446]
        stop <- w450 stop-if-true
        n103 = Greater?(x=w446, y=w445) -> (0:→"Analog":bool)
        n104 = call-poly <vilib>:"DAQmx Read.vi"("task/channels in"=w463, "error in"=w464) -> ("task out"=w460:refnum<k21>, "data"=w458:waveform(dbl)[], "error out"=w452:errorcluster)  [unwired: 11 in]
        n105 = Index Array(array=w458, index=0) -> (element=w456:waveform(dbl))
        n106 = Unbundle By Name(w456) -> ("Y"=w455:dbl[])
        n107 = Array Size(array=w455) -> (size(s)=w448:i32)
        n108 = TDMS Write(0:w462, 5:"Analog Data" ("group name in (Untitled)"), 9:w458, 11:w452) -> (4:w461:refnum<k34>, 15:w449:errorcluster)  [unwired: 2 in, 2 out]
        n109 = Add(x=w448, y=w454) -> (x+y=w453:u32)
        "Analog Samples" <- w453
        n110 = Greater Or Equal?(x=w453, y=w443) -> (x >= y?=w451:bool)
        n111 = local read "stop"() -> (w444:bool)
        n112 = Compound Arithmetic op=OR(w444, w449, w451) -> (w450:bool)
        "Analog Data" <- w450
      }
      n113 = while {
        tunnel: [w567] -> w383
        tunnel: [w550] -> w373
        tunnel: [w576] -> w342
        tunnel: w344 -> [w575]
        tunnel: w345 -> [w574]
        tunnel: w346 -> [w573]
        tunnel: w347 -> [w572]
        shift-right: [w531] -> _
        shift-left: _ -> [w571]
        shift-right: [w570] -> _
        shift-left: u32 0 ("New Lost") -> [w566]
        shift-right: [w569] -> w390
        shift-left: u32[] [] ("NewBuffNum") -> [w559]
        shift-right: [w568] -> w361
        shift-left: u32[] [] ("NewNumLost") -> [w560]
        tunnel: w398 -> [w564]
        tunnel: w336 -> [w554]
        tunnel: w290 -> [w552]
        tunnel: [w550] -> w298
        tunnel: w271 -> [w549]
        tunnel: w296 -> [w546]
        tunnel: w295 -> [w545]
        tunnel: [w546] -> w293
        tunnel: [w545] -> w294
        tunnel: w247 -> [w541]
        tunnel: w246 -> [w540]
        tunnel: w245 -> [w539]
        tunnel: w243 -> [w538]
        tunnel: w241 -> [w537]
        tunnel: w238 -> [w536]
        tunnel: w237 -> [w535]
        tunnel: w236 -> [w534]
        tunnel: [w533] -> w233
        tunnel: [w532] -> w232
        tunnel: w230 -> [w529]
        i -> [w548]
        stop <- w561 stop-if-true
        # "Track Dropped Frames"
        n114 = Greater?(x=w548, y=w549) -> (0:→"Whisk Cam":bool)
        n115 = call <vilib>:"IMAQdx Get Image.vi"("Buffer Number Mode (Next)"=IMAQdx_Buffer_Number_Mode."Next", "error in"=w574, "Image In"=w573, "Session In"=w575) -> ("error out"=w583:errorcluster, "Buffer Number Out"=w531:u32, "Image Out"=w582:T1, "Session Out"=w567:T2)  [unwired: 4 in]
        "Last Whisk Buffer" <- w531
        n116 = case shown="True" w541 {
          selector: w541 -> [w586 _]
          tunnel: w531 -> [_ w596]
          tunnel: w538 -> [_ w595]
          tunnel: w537 -> [_ w594]
          tunnel: w536 -> [_ w593]
          tunnel: w539 -> [_ w590]
          tunnel: [0.0 ("element") w587] -> w543
          tunnel: w540 -> [_ w589]
          tunnel: [w586 w588] -> w542
          frame False {
          }
          frame True {
            n117 = Quotient & Remainder(x=w596, y=w595) -> (x-y*floor(x/y)=w598:dbl, floor(x/y)=w591:dbl)
            n118 = Add(x=w594, y=w593) -> (x+y=w597:dbl)
            n119 = Quotient & Remainder(x=w591, y=w590) -> (x-y*floor(x/y)=w592:dbl)  [unwired: 1 out]
            n120 = In Range and Coerce(upper limit=w597, x=w598, lower limit=w593) -> (In Range?=w588:bool)  [unwired: 1 out]
            n121 = Index Array(array=w589, index=w592) -> (element=w587:dbl)
          }
        }
        n122 = Tick Count (ms)() -> (millisecond timer value=w555:u32)
        n123 = Subtract(x=w555, y=w554) -> (x-y=w558:u32)
        n124 = Add(x=w531, y=w566) -> (x+y=w565:u32)
        n125 = call "IMAQ ImageToArray"("error in (no error)"=w583, "Image"=w582) -> ("error out"=w581:errorcluster, "Image Pixels (U8)"=w580:u8[][])  [unwired: 2 in, 3 out]
        n126 = Multiply(x=w558, y=1.667e-05) -> (x*y=w557:dbl)
        n127 = call <vilib>:"Calculate Frames per Second.vi"("Update Interval (ms)"=u32 2000, "Buffer Number"=w531) -> ("Processed Frames/s"=→"Whisk Cam Fs":dbl)  [unwired: 7 in, 2 out]
        n128 = call "TrackDroppedFrames_2P.vi"("NumLost"=w560, "BuffNum"=w559, "Curr Buffer"=w531, "Prev Lost"=w566, "Prev Buffer"=w571) -> ("New Lost"=w570:u32, "NewNumLost"=w568:u32[], "NewBuffNum"=w569:u32[])  [unwired: 4 in]
        "Dropped" <- w570
        n129 = Greater Or Equal?(x=w565, y=w564) -> (x >= y?=w562:bool)
        n130 = Bundle("Time (min)"=w552, w557) -> (→"Time Elapsed (Min)":cluster{"Time (min)":dbl, dbl})  [unwired: 1 in]
        n131 = Write to Binary File(file (use dialog)=w572, data=w580, error in=w581, 5:FALSE ("prepend array or string size? (T)"), 9:T8."little-endian" ("byte order (0:big-endian, network order)")) -> (refnum out=w576:refnum<file>, error out=w550:errorcluster)  [unwired: 1 in, 1 out]
        n132 = Unbundle By Name(w550) -> ("status"=w563:bool)
        n133 = Compound Arithmetic op=OR(w563, w562, "stop") -> (w561:bool)
        "Whisker Camera" <- w561
        n134 = Replace Array Subset(array=w529, new element=w542, index=w543) -> (w544:bool[])
        "Solenoids" <- w544
        n135 = call-poly <vilib>:"DAQmx Write.vi"("task/channels in"=w535, "data"=w544, "error in"=w534) -> ("task out"=w533:refnum<k21>, "error out"=w532:errorcluster)  [unwired: 10 in, 1 out]
      }
      n136 = while {
        tunnel: w270 -> [w429]
        tunnel: w268 -> [w428]
        tunnel: w269 -> [w432]
        tunnel: w265 -> [w431]
        tunnel: [w427] -> w272
        tunnel: [w433] -> w275
        tunnel: [w431] -> w276
        tunnel: w227 -> [w435]
        tunnel: w226 -> [w434]
        i -> [w436]
        stop <- w423 stop-if-true
        n137 = Tick Count (ms)() -> (millisecond timer value=w440:u32)
        n138 = Subtract(x=w440, y=w434) -> (x-y=w441:u32)
        n139 = Divide(x=w441, y=u32 1000) -> (x/y=w430:dbl)
        n140 = Greater?(x=w435, y=w436) -> (0:→"Web Cam":bool)
        n141 = call "GrabWebCam_2P.vi"("Session In"=w428, "Image In"=w429, "Trial Time"=w430, "AVI Refnum"=w431, "error in"=w432) -> ("Session Out"=w427:T2, "WebCam Img Out"=→"?":T1, "Buffer Number Out"=w425:u32, "error out"=w433:errorcluster)  [unwired: 7 in]
        n142 = call <vilib>:"Calculate Frames per Second.vi"("Update Interval (ms)"=u32 5000, "Buffer Number"=w425) -> ("Processed Frames/s"=→"Web Cam Fs":dbl)  [unwired: 7 in, 2 out]
        n143 = local read "Analog Data"() -> (w424:bool)
        n144 = local read "stop"() -> (w422:bool)
        n145 = Compound Arithmetic op=OR(w422, w424) -> (w423:bool)
      }
      n146 = call <vilib>:"DAQmx Stop Task.vi"("task/channels in"=w294, "error in"=w293) -> ()  [unwired: 12 in, 2 out]
      n147 = Delete From Array(array=w390, length=1, index=0) -> (array with subset deleted=w397:u32[])  [unwired: 1 out]
      n148 = Delete From Array(array=w361, length=1, index=0) -> (array with subset deleted=w396:u32[])  [unwired: 1 out]
      n149 = Close File(refnum=w342, error in=w373) -> (path=w363:path, error out=w364:errorcluster)
      n150 = call <vilib>:"IMAQdx Close Camera.vi"("error in"=w298, "Session In"=w383) -> ()  [unwired: 9 in, 1 out]
      n151 = call <vilib>:"DAQmx Stop Task.vi"("task/channels in"=w358, "error in"=w381) -> ("task out"=w371:refnum<k21>, "error out"=w372:errorcluster)  [unwired: 12 in]
      n152 = call <vilib>:"DAQmx Stop Task.vi"("task/channels in"=w233, "error in"=w232) -> ("task out"=w235:refnum<k21>, "error out"=w234:errorcluster)  [unwired: 12 in]
      n153 = Move(source path=w363, error in=w364, 10:"Target Path") -> (error out=w366:errorcluster)  [unwired: 2 in, 2 out]
      n154 = call <vilib>:"DAQmx Clear Task.vi"("task in"=w371, "error in"=w372) -> ()  [unwired: 13 in, 1 out]
      n155 = Build Array(w397, w396) -> (w394:u32[][])
      n156 = call "IMAQ AVI2 Close"("error in (no error)"=w275, "AVI Refnum"=w276) -> ("error out"=w274:errorcluster)  [unwired: 9 in]
      n157 = call <vilib>:"IMAQdx Close Camera.vi"("error in"=w275, "Session In"=w272) -> ()  [unwired: 9 in, 1 out]
      n158 = call <vilib>:"DAQmx Clear Task.vi"("task in"=w235, "error in"=w234) -> ()  [unwired: 13 in, 1 out]
      n159 = Transpose 2D Array(2D array=w394) -> (transposed array=w395:u32[][])
      n160 = Array To Spreadsheet String(delimiter (Tab)=",", array=w397, 3:"%d" ("format string")) -> (spreadsheet string=w385:string)
      n161 = Array To Spreadsheet String(delimiter (Tab)=",", array=w396, 3:"%d" ("format string")) -> (spreadsheet string=w386:string)
      n162 = call <vilib>:"Simple Error Handler.vi"("error in (no error)"=w366) -> ()  [unwired: 1 in, 8 out]
      n163 = Number To Decimal String(number=w395) -> ()  [unwired: 1 in, 1 out]
      n164 = call <vilib>:"Trim Whitespace.vi"("string"=w385) -> ("trimmed string"=w388:string)  [unwired: 1 in]
      n165 = call <vilib>:"Trim Whitespace.vi"("string"=w386) -> ("trimmed string"=w387:string)  [unwired: 1 in]
      n166 = Move(source path=w218, error in=w274, 10:"Target Path") -> (error out=w273:errorcluster)  [unwired: 2 in, 2 out]
      n167 = Build Array(w388, w387) -> (w389:string[])
      n168 = TDMS Set Properties(5:w389, 7:string[] ["WhiskerCam_DroppedFrameIndex", "WhiskerCam_NumberDropped"] ("channel name(s) in (Untitled)"), 8:w381, 11:w380) -> (0:w382:errorcluster, 3:w384:refnum<k34>)  [unwired: 2 in, 2 out]
      n169 = TDMS Close(8:w382, 11:w384) -> (0:w362:errorcluster, 3:w367:path)
      n170 = Path To String(path=w367) -> (string=w229:string)
      n171 = Concatenate Strings(w229, "_index" ("string")) -> (w368:string)
      n172 = String To Path(string=w368) -> (path=w369:path)
      n173 = TDMS Defragment(4:w362, 7:w367) -> (0:w370:errorcluster)
      n174 = Move(source path=w369, error in=w370, 10:"Target Path") -> ()  [unwired: 2 in, 3 out]
      n175 = Move(source path=w367, error in=w370, 10:"Target Path") -> (error out=w365:errorcluster)  [unwired: 2 in, 2 out]
      n176 = call <vilib>:"Simple Error Handler.vi"("error in (no error)"=w365) -> ()  [unwired: 1 in, 8 out]
      n177 = call <vilib>:"Simple Error Handler.vi"("error in (no error)"=w273) -> ()  [unwired: 1 in, 8 out]
    }
    frame #3 {
      "Complete" <- TRUE ("Data Acquisition - Complete")
    }
  }
